vi "Write Dictionary Elements (Loop).vi"(8 "error in (no error)":errorcluster, 9 "values":variant[](array[variant]), 10 "keys":string[](array[string]), 11 "Control Experiment":refnum<class "SMO.Control Experiment.lvclass">) -> (0 "error out":errorcluster, 3 "Control Experiment out":refnum<class "SMO.Control Experiment.lvclass">)   [LabVIEW 2019, in "SMO.Control Experiment.lvclass"]
uses:
  SMO.Control Experiment.lvclass
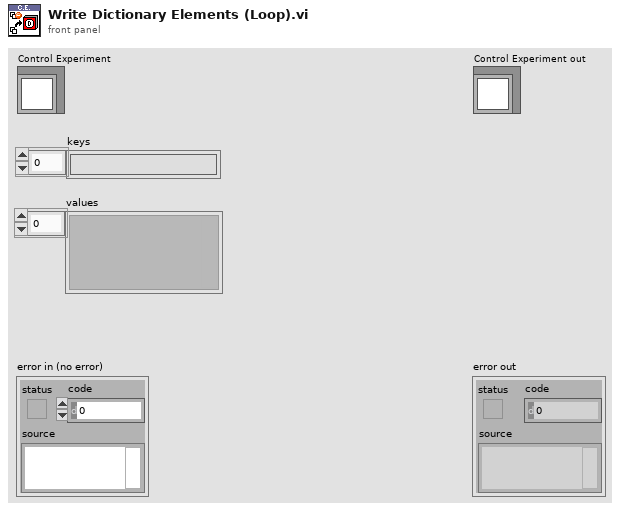
[diagram p1: front panel]
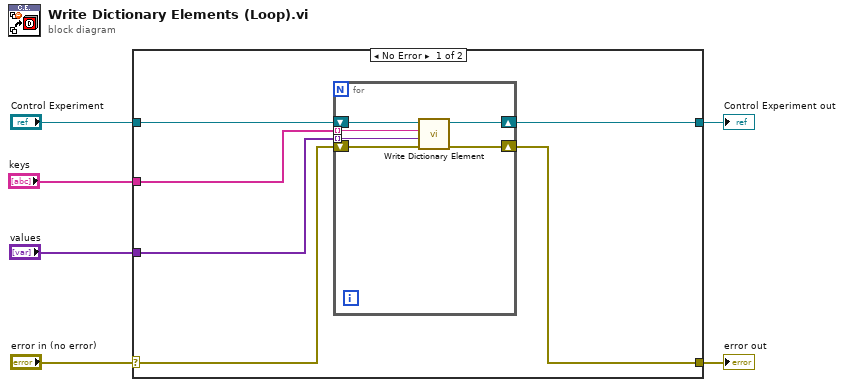
[diagram p0: block diagram]
diagram:
  n1 = case shown="No Error" "error in (no error)" {
    selector: "error in (no error)" -> [w10 w19]
    tunnel: [w7 w19] -> w5
    tunnel: [w11 w20] -> w3
    tunnel: "Control Experiment" -> [w12 w20]
    tunnel: "keys" -> [w8 _]
    tunnel: "values" -> [w9 _]
    frame No Error {
      n2 = for {
        shift-right: [w17] -> w11
        shift-left: w12 -> [w18]
        shift-right: [w15] -> w7
        shift-left: w10 -> [w16]
        tunnel: w8 -> [w14] mode=indexing
        tunnel: w9 -> [w13] mode=indexing
        n3 = call "Write Dictionary Element.vi"("error in (no error)"=w16, "value"=w13, "key"=w14, "Control Experiment"=w18) -> ("error out"=w15:errorcluster, "Control Experiment out"=w17:refnum<class "SMO.Control Experiment.lvclass">)  [unwired: 6 in]
      }
    }
    frame Error {
    }
  }
  "error out" <- w5
  "Control Experiment out" <- w3
